vi "Get Pattern Data.vi"(9 "File Name":i32[](array[numeric]), 10 "Folder Name":string, 11 "Dispense.lvclass":refnum<class "Dispense.lvclass">) -> (3 "Dispense Out":refnum<class "Dispense.lvclass">)   [LabVIEW 2020, in "Dispense.lvclass"]
uses:
  Dispense.lvclass
  Dispense.lvclass/Dispense.ctl
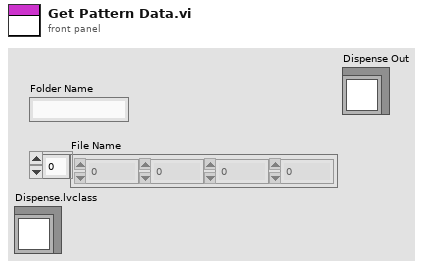
[diagram p1: front panel]
types:
  T1 = cluster{"Time To Go Down":i32, "Time to Dispense":i32}[]
  T2 = cluster{"Time To Go Down":i32, "Time to Dispense":i32}
  T3 = typedef "File Paths.ctl" = cluster{"Glue Pattern Folder":path, "Carrier Tray Folder":path, "Pick Up Tool Fixture Folder":path, "Components Folder":path, "Bellows Tool Offset.txt":path, "Pick Up Tool Offset.txt":path, "Dispense Tip Offset.txt":path, "Log Files":path}
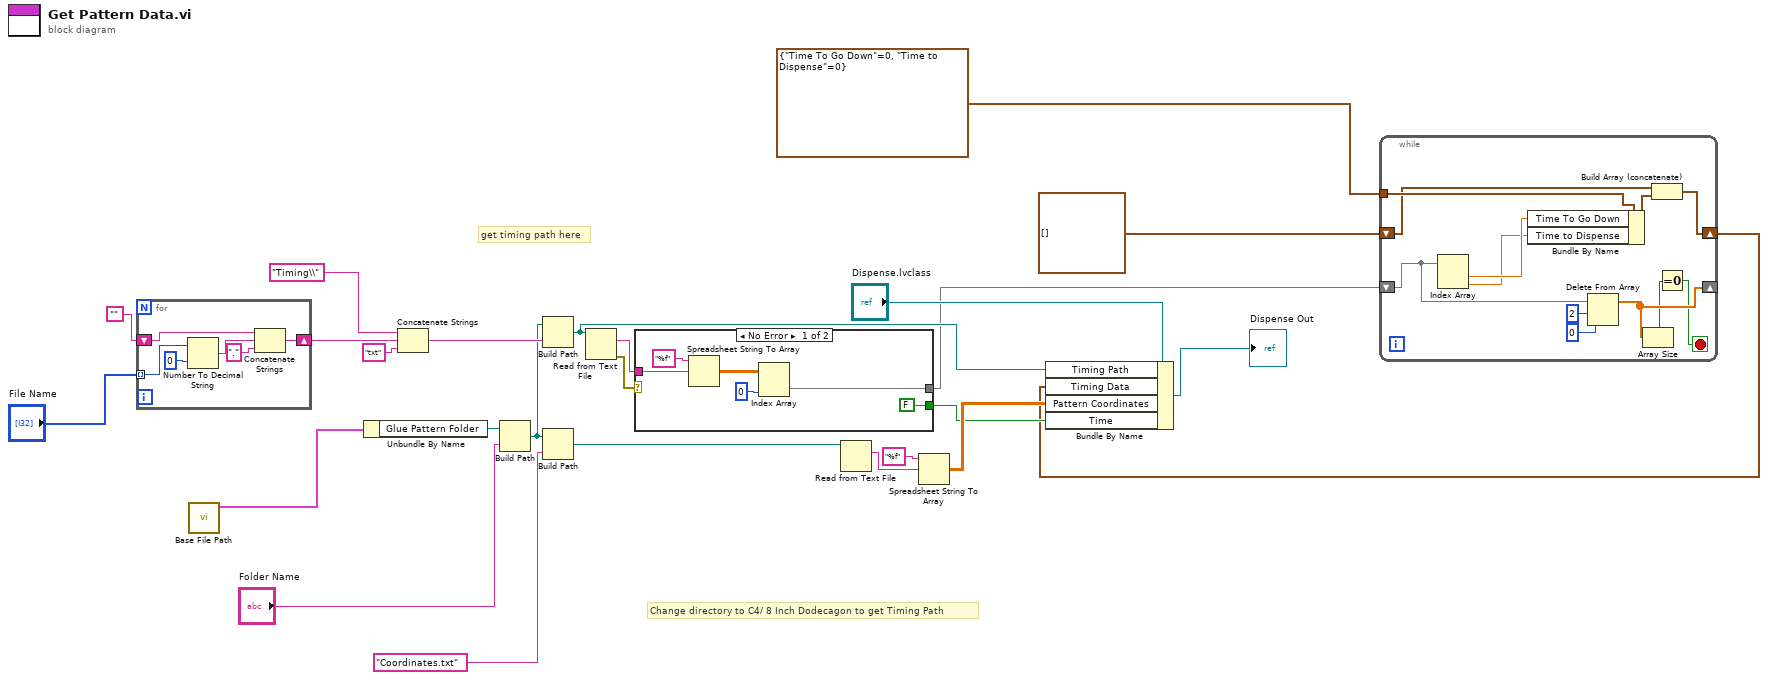
[diagram p0: block diagram]
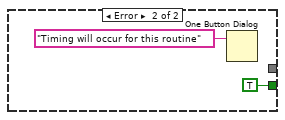
[diagram p2: hidden frame]
diagram:
  # "Change directory to C4/ 8 Inch Dodecagon to get Timing Path"
  # "get timing path here"
  n1 = for {
    tunnel: "File Name" -> [w31] mode=indexing
    shift-right: [w27] -> w21
    shift-left: "" -> [w26]
    n2 = Number To Decimal String(number=w31, width (-)=i16 0) -> (decimal integer string=w29:string)
    n3 = Concatenate Strings(w26, w29, "." ("string")) -> (w27:string)
  }
  n4 = call "Base File Path.vi"() -> ("Paths Out"=w12:T3)  [unwired: 11 in]
  n5 = Unbundle By Name(w12) -> ("Glue Pattern Folder"=w16:path)
  n6 = Concatenate Strings("Timing\\" ("name or relative path"), w21, "txt" ("string")) -> (w24:string)
  n7 = Build Path(base path=w16, name or relative path="Folder Name") -> (appended path=w23:path)
  n8 = Build Path(base path=w23, name or relative path=w24) -> (appended path=w10:path)
  n9 = Build Path(base path=w23, name or relative path="Coordinates.txt") -> (appended path=w18:path)
  n10 = Read from Text File(file (use dialog)=w10) -> (text=w25:string, error out=w5:errorcluster)  [unwired: 3 in, 2 out]
  n11 = case shown="No Error" w5 {
    tunnel: w25 -> [w36 _]
    tunnel: [w34 _] -> w4
    tunnel: [FALSE TRUE] -> w8
    frame No Error {
      n12 = Spreadsheet String To Array(format string="%f", spreadsheet string=w36) -> (array=w35:dbl[][])  [unwired: 2 in]
      n13 = Index Array(array=w35, index (col)=0 ("disabled index (col)")) -> (element=w34:dbl[])  [unwired: 1 in]
    }
    frame Error {
      n14 = One Button Dialog(message="Timing will occur for this routine") -> ()  [unwired: 1 in, 1 out]
    }
  }
  n15 = Read from Text File(file (use dialog)=w18) -> (text=w14:string)  [unwired: 3 in, 3 out]
  n16 = Spreadsheet String To Array(format string="%f", spreadsheet string=w14) -> (array=w9:dbl[][])  [unwired: 2 in]
  n17 = while {
    shift-right: [w42] -> _
    shift-left: w4 -> [w49]
    shift-right: [w43] -> w1
    shift-left: T1 [] -> [w44]
    tunnel: T2 {"Time To Go Down"=0, "Time to Dispense"=0} -> [w46]
    stop <- w40 stop-if-true
    n18 = Index Array(array=w49) -> (element #1=w51:dbl, element #2=w50:dbl)  [unwired: 2 in]
    n19 = Bundle By Name(cluster=w46, "Time To Go Down"=w51, "Time to Dispense"=w50) -> (w45:T2)
    n20 = Delete From Array(array=w49, length=2, index=0) -> (array with subset deleted=w42:dbl[])  [unwired: 1 out]
    n21 = Array Size(array=w42) -> (size(s)=w41:i32)
    n22 = Build Array (concatenate)(w44, w45) -> (w43:T1)
    n23 = Equal To 0?(x=w41) -> (x = 0?=w40:bool)
  }
  n24 = Bundle By Name(cluster="Dispense.lvclass", "Timing Path"=w10, "Timing Data"=w1, "Pattern Coordinates"=w9, "Time"=w8) -> (→"Dispense Out":refnum<class "Dispense.lvclass">)
